vi "InitializeMissionArrays.vi"() -> (2 "Mission Points of Interest":T1[](array[typedef]) {"North" format="%#_10f"; "East" format="%#_8f"}, 3 "Initialized Mission Arrays":T2 {"Readable Missions"."Points of Interest"."North" format="%#_10f"; "Readable Missions"."Points of Interest"."East" format="%#_8f"})   [LabVIEW 2013]
doc: "This initializes the arrays that are used for mission tracking and packs them into a cluster. It also initializes an empty UTM array for wiping points of interest in the future.\n\nEric Schneider, August 2014"
uses:
  TypeDef/mission_arrays.ctl
  cRIO_Code/Data/TypeDefs/MissionDescription.ctl
  cRIO_Code/Data/TypeDefs/MissionTypeControl.ctl
  cRIO_Code/Data/TypeDefs/UTM Location.ctl
  cRIO_Code/Logic/Classes/Missions/GenericMission/GenericMission.lvclass
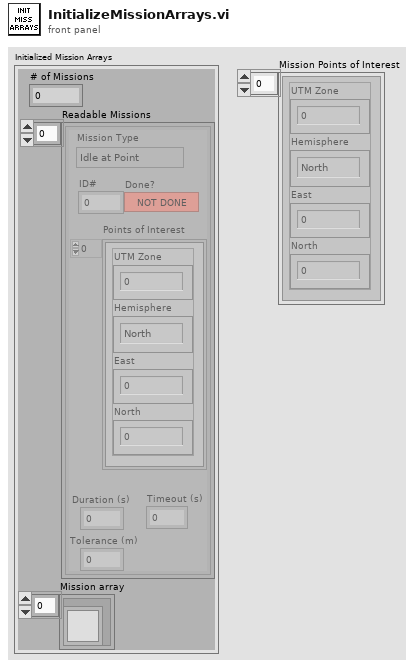
[diagram p1: front panel]
types:
  T1 = typedef "UTM Location.ctl" = cluster{"UTM Zone":dbl, "Hemisphere":enum16{"North", "South"}, "East":dbl, "North":dbl}
  T2 = typedef "mission_arrays.ctl" = cluster{"# of Missions":i32, "Readable Missions":T3[], "Mission array":refnum<class "GenericMission.lvclass">[]}
  T3 = typedef "MissionDescription.ctl" = cluster{"Duration (s)":dbl, "Timeout (s)":dbl, "Tolerance (m)":dbl, "Mission Type":T4, "Points of Interest":T1[], "ID#":i32, "Done?":bool}
  T4 = typedef "MissionTypeControl.ctl" = enum16{"Idle at Point", "Drive to Waypoint", "Round Buoy to Port", "Round Buoy to Starboard", "Pass Between Buoys", "Station Keeping"}
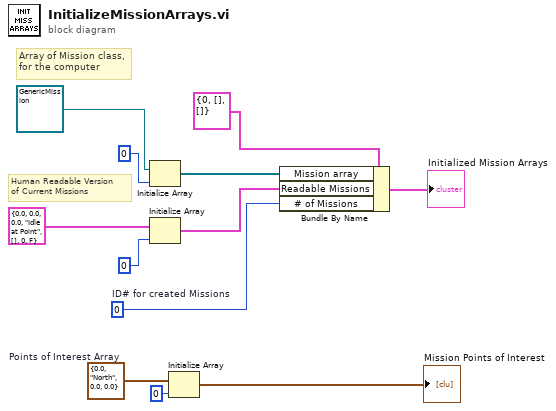
[diagram p0: block diagram]
diagram:
  w3 = T1 {"UTM Zone"=0.0, "Hemisphere"=enum."North", "East"=0.0, "North"=0.0}  # Points of Interest Array
  w7 = 0  # ID# for created Missions
  # "Array of Mission class, for the computer"
  # "Human Readable Version\nof Current Missions"
  n1 = Initialize Array "Initialize Array"(refnum<class "GenericMission.lvclass"> refnum ("GenericMission.lvclass"), 0 ("dimension size")) -> (w5:refnum<class "GenericMission.lvclass">[])
  n2 = Initialize Array "Initialize Array"(T3 {"Duration (s)"=0.0, "Timeout (s)"=0.0, "Tolerance (m)"=0.0, "Mission Type"=enum."Idle at Point", "Points of Interest"=[], "ID#"=0, "Done?"=FALSE} ("input cluster"), 0 ("dimension size")) -> (w6:T3[])
  n3 = Initialize Array(w3, 0 ("dimension size")) -> (→"Mission Points of Interest":T1[])
  n4 = Bundle By Name(cluster=T2 {"# of Missions"=0, "Readable Missions"=[], "Mission array"=[]} ("Cluster"), "Mission array"=w5, "Readable Missions"=w6, "# of Missions"=w7) -> (→"Initialized Mission Arrays":T2)
